vi "Read latest Position.vi"(8 "error in (no error)":errorcluster, 11 "Fine SIM Motion Controller in":refnum<class "Fine SIM Motion Controller.lvclass">) -> (0 "error out":errorcluster, 2 "Current Position":dbl, 3 "Fine SIM Motion Controller out":refnum<class "Fine SIM Motion Controller.lvclass">)   [LabVIEW 2022 SP3, in "Fine SIM Motion Controller.lvclass"]
uses:
  Fine SIM Motion Controller.lvclass
  C:/Stage-Work/MAS/Axis Objects/Motion Controller/Parent SIM Motion Controller.lvclass
  Motion Controller/Parent SIM Motion Controller.lvclass/Parent SIM Motion Controller.ctl
  Motion Controller/Accessors/Read Sim Axis Data.vi
  Motion Controller/Accessors/Write Sim Axis Data.vi
  Fine SIM Motion Controller.lvclass/Fine SIM Motion Controller.ctl
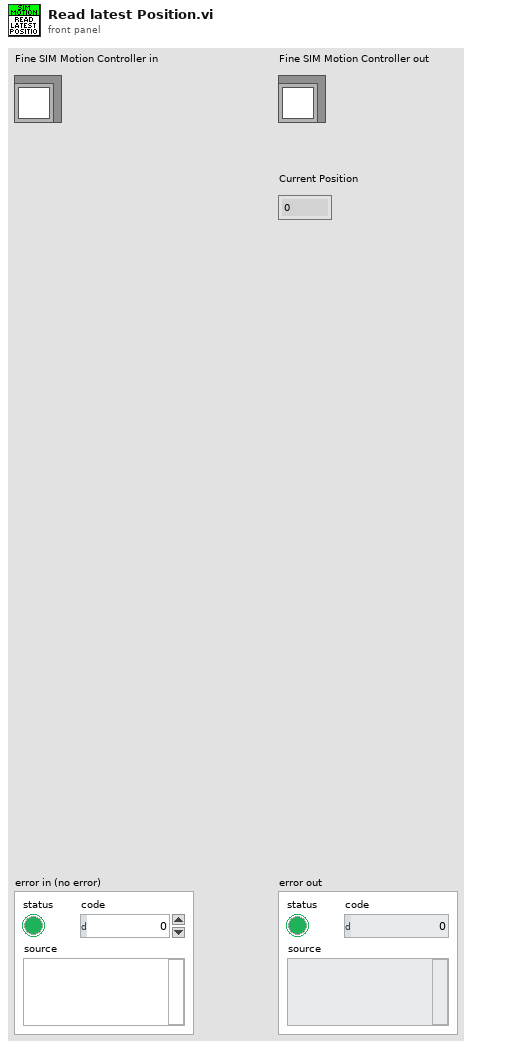
[diagram p1: front panel]
types:
  T1 = typedef "Parent SIM Motion Controller.lvclass/Axis Data.ctl" = cluster{"Axis Parameters":T2, "Axis Settings":T4, "Time Stamp":timestamp}
  T2 = typedef "Parent SIM Motion Controller.lvclass/Axis Parameters.ctl" = cluster{"Moving":bool, "Homed":bool, "Desired Position":dbl, "Current Positon":dbl, "Current Speed":dbl, "Home Status":T3}
  T3 = typedef "Parent SIM Motion Controller.lvclass/Homing Status.ctl" = enum16{"Inital Home Motion", "Final Home Motion"}
  T4 = typedef "Parent SIM Motion Controller.lvclass/Axis Settings.ctl" = cluster{"Speed":dbl, "Acceleration":dbl}
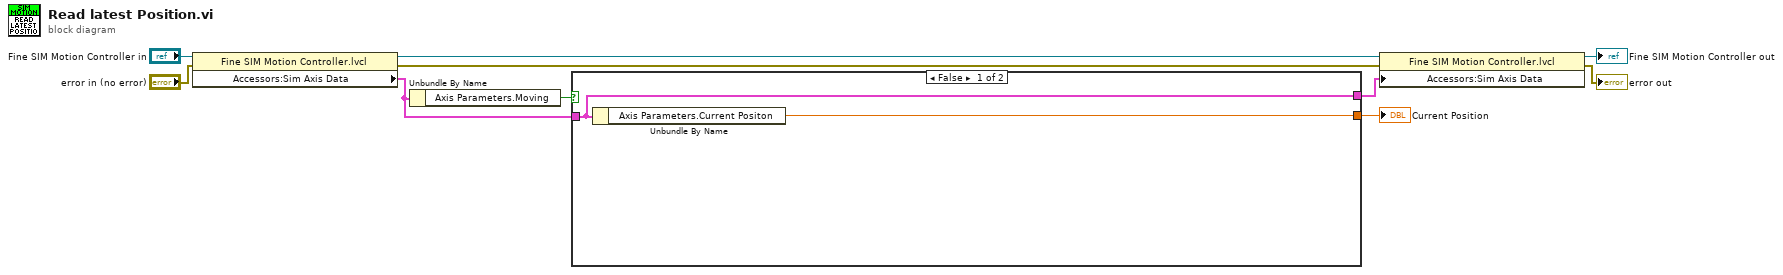
[diagram p0: block diagram]
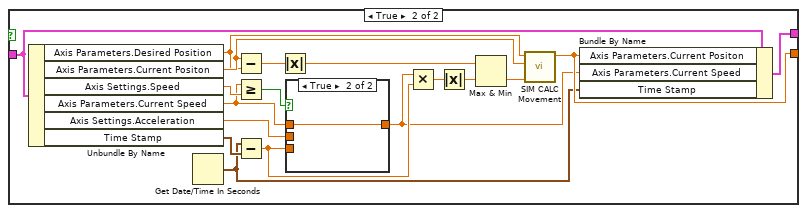
[diagram p2: hidden frame]
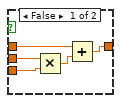
[diagram p3: hidden frame]
diagram:
  n1 = property class="Fine SIM Motion Controller.lvcl"(reference="Fine SIM Motion Controller in", error in="error in (no error)") -> (reference out=w3:refnum<class "Fine SIM Motion Controller.lvclass">, error out=w7:errorcluster, "Accessors:Sim Axis Data"=w9:T1)
  n2 = Unbundle By Name(w9) -> ("Axis Parameters.Moving"=w8:bool)
  n3 = case shown="False" w8 {
    tunnel: w9 -> [w12 w30]
    tunnel: [w12 w28] -> w1
    tunnel: [w11 w29] -> w10
    frame False {
      n4 = Unbundle By Name(w12) -> ("Axis Parameters.Current Positon"=w11:dbl)
    }
    frame True {
      n5 = Unbundle By Name(w30) -> ("Axis Parameters.Desired Position"=w18:dbl, "Axis Parameters.Current Positon"=w19:dbl, "Axis Settings.Speed"=w25:dbl, "Axis Parameters.Current Speed"=w24:dbl, "Axis Settings.Acceleration"=w23:dbl, "Time Stamp"=w21:timestamp)
      n6 = Get Date/Time In Seconds() -> (seconds since 1Jan1904=w20:timestamp)
      n7 = Subtract(x=w19, y=w18) -> (x-y=w17:dbl)
      n8 = Greater Or Equal?(x=w24, y=w25) -> (x >= y?=w26:bool)
      n9 = Subtract(x=w20, y=w21) -> (x-y=w27:dbl)
      n10 = Absolute Value(x=w17) -> (abs(x)=w15:dbl)
      n11 = case shown="True" w26 {
        tunnel: [w31 w36] -> w22
        tunnel: w24 -> [w32 w36]
        tunnel: w27 -> [w35 _]
        tunnel: w23 -> [w34 _]
        frame False {
          n12 = Multiply(x=w34, y=w35) -> (x*y=w33:dbl)
          n13 = Add(x=w32, y=w33) -> (x+y=w31:dbl)
        }
        frame True {
        }
      }
      n14 = Multiply(x=w22, y=w27) -> (x*y=w16:dbl)
      n15 = Absolute Value(x=w16) -> (abs(x)=w14:dbl)
      n16 = Max & Min(x=w15, y=w14) -> (min(x,y)=w13:dbl)  [unwired: 1 out]
      n17 = call "SIM CALC Movement.vi"("New Distance"=w13, "Current"=w19, "Desired"=w18) -> ("New Current"=w29:dbl)  [unwired: 8 in]
      n18 = Bundle By Name(cluster=w30, "Axis Parameters.Current Positon"=w29, "Axis Parameters.Current Speed"=w22, "Time Stamp"=w20) -> (w28:T1)
    }
  }
  "Current Position" <- w10
  n19 = property class="Fine SIM Motion Controller.lvcl"(reference=w3, error in=w7, "Accessors:Sim Axis Data"=w1) -> (reference out=→"Fine SIM Motion Controller out":refnum<class "Fine SIM Motion Controller.lvclass">, error out=→"error out":errorcluster)
